vi "Test.vi"() -> ()   [LabVIEW 2012]
doc: "This VI is called when test mode begins, and will automatically be terminated when it ends. You can add manual or automatic tests and invoke them from the dashboard."
uses:
  Robot Global Data.vi
panel:
  out "error out":errorcluster
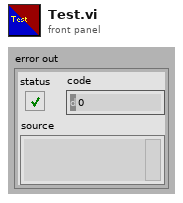
[diagram p1: front panel]
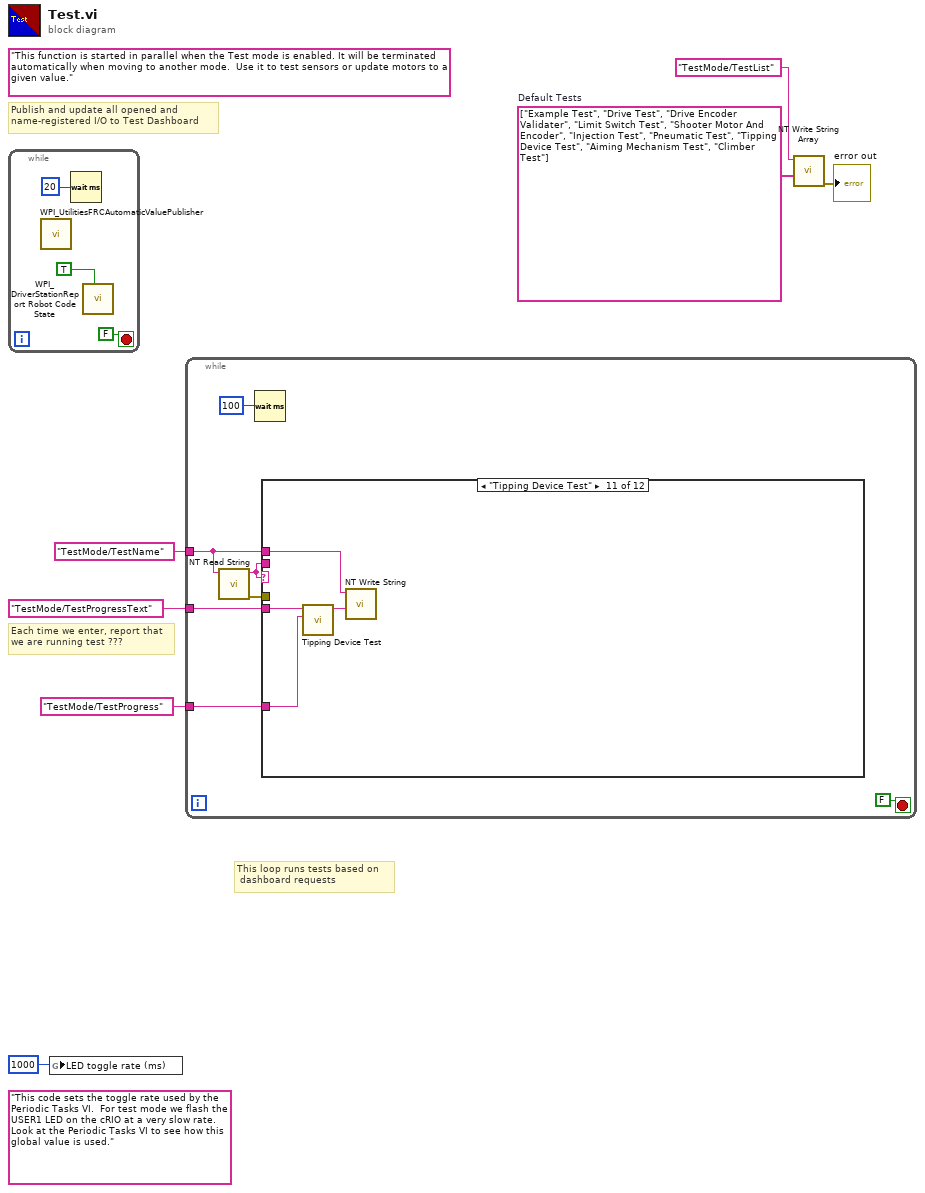
[diagram p0: block diagram]
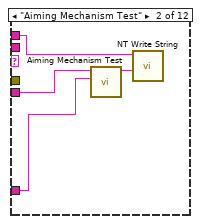
[diagram p3: hidden frame]
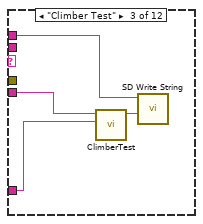
[diagram p4: hidden frame]
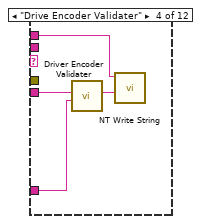
[diagram p5: hidden frame]
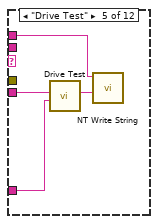
[diagram p6: hidden frame]
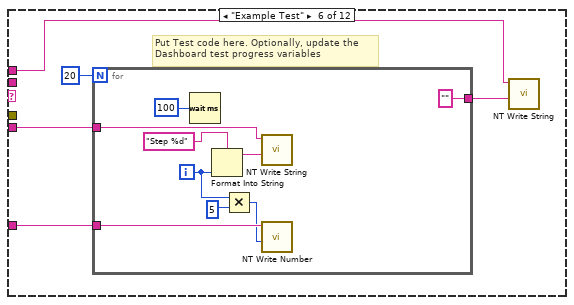
[diagram p7: hidden frame]
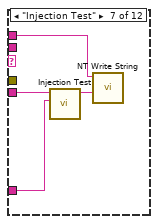
[diagram p8: hidden frame]
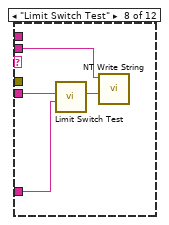
[diagram p9: hidden frame]
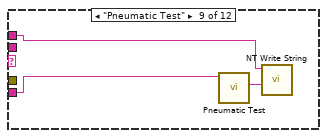
[diagram p10: hidden frame]
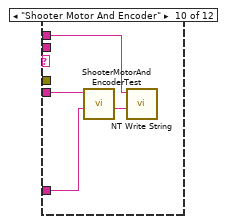
[diagram p11: hidden frame]
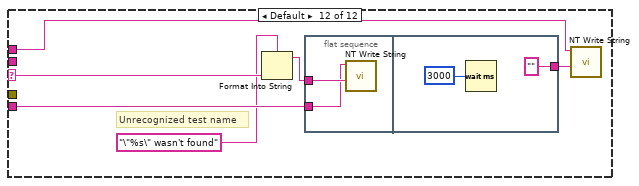
[diagram p12: hidden frame]
diagram:
  w3 = string[] ["Example Test", "Drive Test", "Drive Encoder Validater", "Limit Switch Test", "Shooter Motor And Encoder", "Injection Test", "Pneumatic Test", "Tipping Device Test", "Aiming Mechanism Test", "Climber Test"]  # Default Tests
  (unwired) "This code sets the toggle rate used by the Periodic Tasks VI.  For test mode we flash the USER1 LED on the cRIO at a very slow rate.  Look at the Periodic Tasks VI to see how this global value is used."
  (unwired) "This function is started in parallel when the Test mode is enabled. It will be terminated automatically when moving to another mode.  Use it to test sensors or update motors to a given value."
  # "This loop runs tests based on \n dashboard requests"
  # "Publish and update all opened and\nname-registered I/O to Test Dashboard"
  # "Each time we enter, report that\nwe are running test ???"
  n1 = while {
    stop <- FALSE stop-if-true
    n2 = call "WPI_UtilitiesFRCAutomaticValuePublisher.vi"() -> ()  [unwired: 12 in]
    n3 = Wait (ms)(milliseconds to wait=u32 20) -> ()  [unwired: 1 out]
    n4 = call <vilib>:"WPI_DriverStationReport Robot Code State.vi"("Test"=TRUE ("Autonomous")) -> ()  [unwired: 10 in, 1 out]
  }
  n5 = global write "Robot Global Data.vi" "LED toggle rate (ms)"(u32 1000 ("LED ms toggle rate")) -> ()
  n6 = while {
    tunnel: "TestMode/TestName" ("Name") -> [w12]
    tunnel: "TestMode/TestProgressText" ("Name") -> [w15]
    tunnel: "TestMode/TestProgress" ("Name") -> [w14]
    stop <- FALSE stop-if-true
    n7 = call <vilib>:"NT Read String.vi"("Name"=w12) -> ("error out"=w11:errorcluster, "String"=w13:string)  [unwired: 9 in]
    n8 = Wait (ms)(milliseconds to wait=u32 100) -> ()  [unwired: 1 out]
    n9 = case shown="\"Tipping Device Test\"" w13 {
      selector: w13 -> [_ _ _ _ _ _ _ _ _ _ _ w71]
      tunnel: w12 -> [_ w19 w23 w26 w31 w34 w48 _ w57 w59 w65 w68]
      tunnel: w15 -> [_ w21 w25 w29 w33 w37 w51 w54 w56 w61 w64 w72]
      tunnel: w14 -> [_ w20 w24 w28 w32 w38 w50 w53 _ w62 w63 _]
      tunnel: w13 -> [_ _ _ _ _ _ _ w55 _ _ _ _]
      tunnel: w11 -> [_ _ _ _ _ _ _ _ _ _ _ _]
      frame "", " " {
        # "No test to run"
      }
      frame "Aiming Mechanism Test" {
        n10 = call "Aiming Mechanism Test.vi"("progress"=w20, "progressText"=w21) -> ("endTestText"=w18:string)  [unwired: 9 in]
        n11 = call <vilib>:"NT Write String.vi"("String"=w18, "Name"=w19) -> ()  [unwired: 9 in, 1 out]
      }
      frame "Climber Test" {
        n12 = call "ClimberTest.vi"("progress"=w24, "progressText"=w25) -> ("endTestText"=w22:string)  [unwired: 9 in]
        n13 = call <vilib>:"SD Write String.vi"("String"=w22, "Name"=w23) -> ()  [unwired: 8 in, 2 out]
      }
      frame "Drive Encoder Validater" {
        n14 = call "Driver Encoder Validater.vi"("Progress"=w28, "ProgressText"=w29) -> ("EndTestText"=w27:string)  [unwired: 8 in]
        n15 = call <vilib>:"NT Write String.vi"("String"=w27, "Name"=w26) -> ()  [unwired: 9 in, 1 out]
      }
      frame "Drive Test" {
        n16 = call "Drive Test.vi"("Progress"=w32, "ProgressText"=w33) -> ("EndTestText"=w30:string)  [unwired: 9 in]
        n17 = call <vilib>:"NT Write String.vi"("String"=w30, "Name"=w31) -> ()  [unwired: 9 in, 1 out]
      }
      frame "Example Test" {
        # "Put Test code here. Optionally, update the\nDashboard test progress variables"
        n18 = for {
          N: 20 -> [_]
          tunnel: w38 -> [w47]
          tunnel: w37 -> [w45]
          tunnel: ["" ("String")] -> w35
          i -> [w42]
          n19 = Wait (ms)(milliseconds to wait=u32 100) -> ()  [unwired: 1 out]
          n20 = Format Into String(format string="Step %d", w42) -> (resulting string=w40:string)  [unwired: 2 in, 1 out]
          n21 = Multiply(x=w42, y=u32 5 ("milliseconds to wait")) -> (x*y=w43:u32)
          n22 = call <vilib>:"NT Write String.vi"("String"=w40, "Name"=w45) -> ()  [unwired: 9 in, 1 out]
          n23 = call <vilib>:"NT Write Number.vi"("Numeric"=w43, "Name"=w47) -> ()  [unwired: 9 in, 1 out]
        }
        n24 = call <vilib>:"NT Write String.vi"("String"=w35, "Name"=w34) -> ()  [unwired: 9 in, 1 out]
      }
      frame "Injection Test" {
        n25 = call "Injection Test.vi"("Progress"=w50, "ProgressText"=w51) -> ("EndTestText"=w49:string)  [unwired: 9 in]
        n26 = call <vilib>:"NT Write String.vi"("String"=w49, "Name"=w48) -> ()  [unwired: 9 in, 1 out]
      }
      frame "Limit Switch Test" {
        n27 = call "Limit Switch Test.vi"("Progress"=w53, "ProgressText"=w54) -> ("EndTestText"=w52:string)  [unwired: 9 in]
        n28 = call <vilib>:"NT Write String.vi"("String"=w52, "Name"=w55) -> ()  [unwired: 9 in, 1 out]
      }
      frame "Pneumatic Test" {
        n29 = call "Pneumatic Test.vi"("ProgressText"=w56) -> ("EndTestText"=w58:string)  [unwired: 10 in]
        n30 = call <vilib>:"NT Write String.vi"("String"=w58, "Name"=w57) -> ()  [unwired: 9 in, 1 out]
      }
      frame "Shooter Motor And Encoder" {
        n31 = call "ShooterMotorAndEncoderTest.vi"("Progress"=w62, "ProgressText"=w61) -> ("EndTestText"=w60:string)  [unwired: 9 in]
        n32 = call <vilib>:"NT Write String.vi"("String"=w60, "Name"=w59) -> ()  [unwired: 9 in, 1 out]
      }
      frame "Tipping Device Test" {
        n33 = call "Tipping Device Test.vi"("Progress"=w63, "ProgressText"=w64) -> ("EndTestText"=w66:string)  [unwired: 9 in]
        n34 = call <vilib>:"NT Write String.vi"("String"=w66, "Name"=w65) -> ()  [unwired: 9 in, 1 out]
      }
      frame Default {
        # "Unrecognized test name"
        n35 = Format Into String(format string="\"%s\" wasn't found" ("Name"), w71) -> (resulting string=w70:string)  [unwired: 2 in, 1 out]
        n36 = flat-sequence {
          tunnel: w72 -> [w73]
          tunnel: w70 -> [w74]
          tunnel: ["" ("Name")] -> w67
          frame #0 {
            n37 = call <vilib>:"NT Write String.vi"("String"=w74, "Name"=w73) -> ()  [unwired: 9 in, 1 out]
          }
          frame #1 {
            n38 = Wait (ms)(milliseconds to wait=u32 3000) -> ()  [unwired: 1 out]
          }
        }
        n39 = call <vilib>:"NT Write String.vi"("String"=w67, "Name"=w68) -> ()  [unwired: 9 in, 1 out]
      }
    }
  }
  n40 = call <vilib>:"NT Write String Array.vi"("String Array"=w3, "Name"="TestMode/TestList") -> ("error out"=→"error out":errorcluster)  [unwired: 9 in]
